vi "Initialize-object.vi"(8 "error in (no error)":errorcluster, 9 "DOTNET settings":T1={"Target IP"="128.178.146.163", "Target broadcast port"=11000, "Target communication port"=-1, "clientID"=-1, "Broadcast IP"="224.168.100.2", "Servercount"=-1, "Device IDs"=[]}, 10 "TCP settings":T3={"Target IP"="128.178.146.163", "Target TCP port"=12500, "TCP read mode"=enum."CRLF", "TCP read buffer"=4096, "Read timeout"=5000}) -> (0 "error out":errorcluster, 3 "SM1000-control out":T4)   [LabVIEW 2013, in "EC1000-control.lvlib" / "SM1000-control.lvclass"]
uses:
  SM1000-control.lvclass
  Object-reference.ctl
  TCP-settings.ctl
  DOTNET-settings.ctl
  Device-identification.ctl
  DOTNET-status.ctl
  SM1000-control.lvclass/SM1000-control.ctl
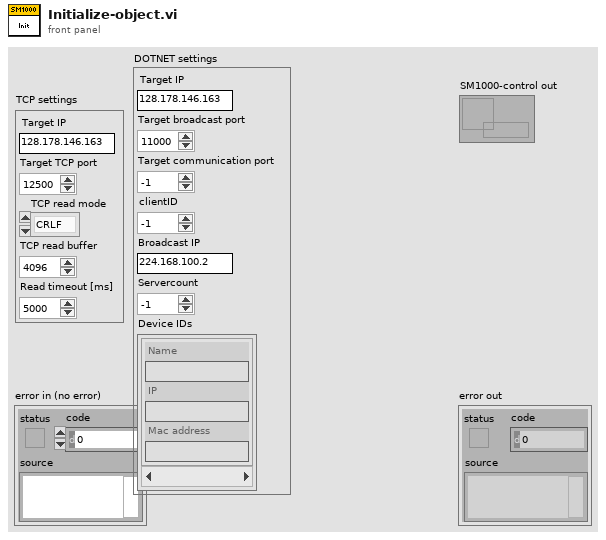
[diagram p1: front panel]
types:
  T1 = typedef "EC1000-control.lvlib/SM1000-control.lvclass/DOTNET-settings.ctl" = cluster{"Target IP":string, "Target broadcast port":i32, "Target communication port":i32, "clientID":i32, "Broadcast IP":string, "Servercount":i32, "Device IDs":T2[]}
  T2 = typedef "EC1000-control.lvlib/SM1000-control.lvclass/Device-identification.ctl" = cluster{"Name":string, "IP":string, "Mac address":string}
  T3 = typedef "EC1000-control.lvlib/SM1000-control.lvclass/TCP-settings.ctl" = cluster{"Target IP":string, "Target TCP port":u16, "TCP read mode":enum16{"Standard", "Buffered", "CRLF", "Immediate"}, "TCP read buffer":i32, "Read timeout":i32}
  T4 = typedef "EC1000-control.lvlib/SM1000-control.lvclass/Object-reference.ctl" = refnum<data-value>
  T5 = typedef "EC1000-control.lvlib/SM1000-control.lvclass/DOTNET-status.ctl" = cluster{"LECBroadcast":bool, "LECSession":bool, "CommonLib":bool, "CtiTelnet":bool, "FTPClient":bool, "ECUtils":bool}
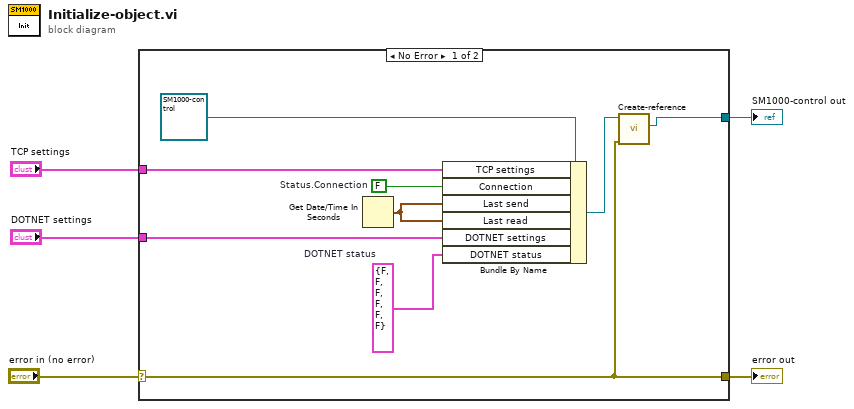
[diagram p0: block diagram]
diagram:
  n1 = case shown="No Error" "error in (no error)" {
    selector: "error in (no error)" -> [w11 w15]
    tunnel: [w11 w15] -> w4
    tunnel: [w8 _] -> w3
    tunnel: "TCP settings" -> [w14 _]
    tunnel: "DOTNET settings" -> [w7 _]
    frame No Error {
      w6 = T5 {"LECBroadcast"=FALSE, "LECSession"=FALSE, "CommonLib"=FALSE, "CtiTelnet"=FALSE, "FTPClient"=FALSE, "ECUtils"=FALSE}  # DOTNET status
      w13 = FALSE  # Status.Connection
      n2 = Get Date/Time In Seconds() -> (seconds since 1Jan1904=w12:timestamp)
      n3 = Bundle By Name(cluster=refnum<class "SM1000-control.lvclass"> refnum ("EC1000-control.lvlib:SM1000-control.lvclass"), "TCP settings"=w14, "Connection"=w13, "Last send"=w12, "Last read"=w12, "DOTNET settings"=w7, "DOTNET status"=w6) -> (w9:refnum<class "SM1000-control.lvclass">)
      n4 = call "Create-reference.vi"("error in (no error)"=w11, "SM1000-control in"=w9) -> ("Object reference"=w8:T4)  [unwired: 7 in, 2 out]
    }
    frame Error {
    }
  }
  "error out" <- w4
  "SM1000-control out" <- w3
